vi "4_bit_adder.vi"(0 "A3":bool, 1 "A2":bool, 2 "A1":bool, 3 "A0":bool, 11 "B3":bool, 12 "B2":bool, 13 "B1":bool, 14 "B0":bool) -> (4 "Y4":bool, 6 "Y3":bool, 7 "Somma decimale":dbl, 8 "Y2":bool, 10 "Y1":bool, 15 "Y0":bool)   [LabVIEW 2024]
doc: "Effettua la somma tra 2 numeri binari (di massimo 4 bit ognuno) e ne restituisce la somma in binario e in valore decimale."
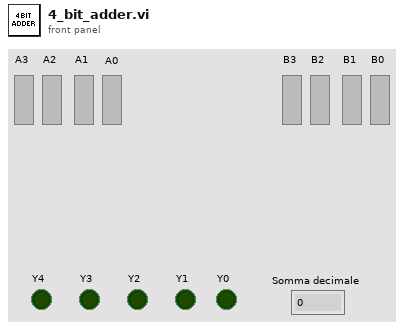
[diagram p1: front panel]
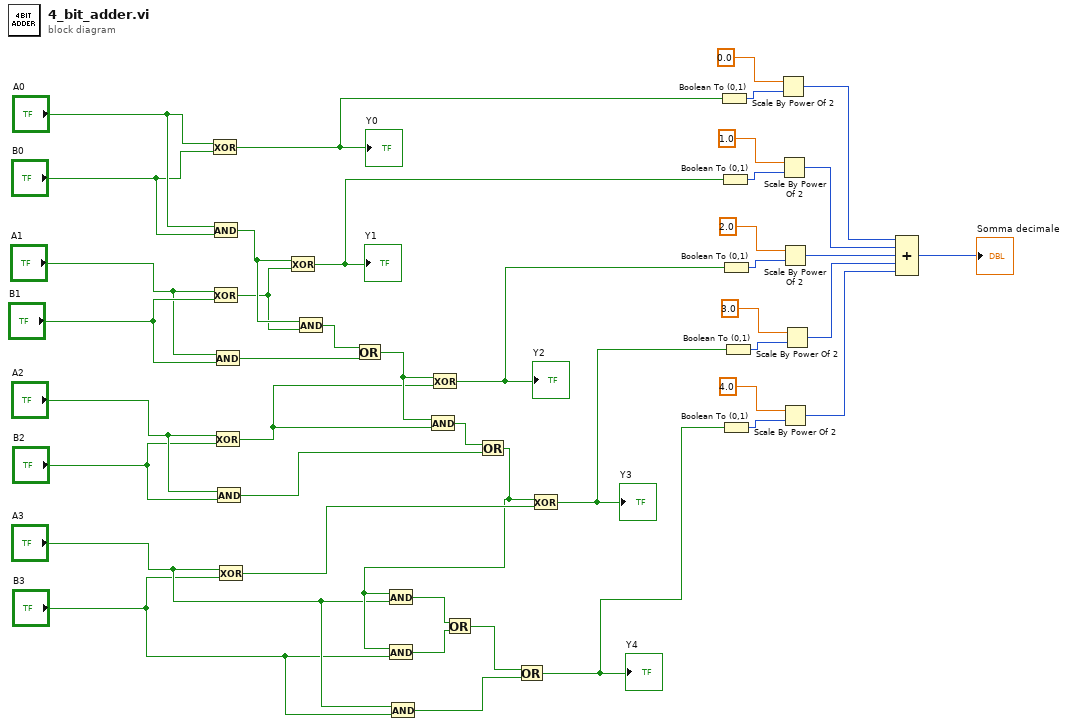
[diagram p0: block diagram]
diagram:
  n1 = Exclusive Or(1:"B0", 2:"A0") -> (0:w5:bool)
  "Y0" <- w5
  n2 = And(x="A0", y="B0") -> (x .and. y?=w39:bool)
  n3 = Exclusive Or(1:"B1", 2:"A1") -> (0:w38:bool)
  n4 = And(x="A1", y="B1") -> (x .and. y?=w37:bool)
  n5 = Exclusive Or(1:"B2", 2:"A2") -> (0:w32:bool)
  n6 = And(x="A2", y="B2") -> (x .and. y?=w30:bool)
  n7 = Exclusive Or(1:"B3", 2:"A3") -> (0:w29:bool)
  n8 = Exclusive Or(1:w38, 2:w39) -> (0:w4:bool)
  "Y1" <- w4
  n9 = And(x=w39, y=w38) -> (x .and. y?=w36:bool)
  n10 = Or(x=w36, y=w37) -> (x .or. y?=w33:bool)
  n11 = And(x="A3", y="B3") -> (x .and. y?=w27:bool)
  n12 = And(x=w33, y=w32) -> (x .and. y?=w31:bool)
  n13 = Exclusive Or(1:w32, 2:w33) -> (0:w3:bool)
  "Y2" <- w3
  n14 = Or(x=w31, y=w30) -> (x .or. y?=w24:bool)
  n15 = And(x=w24, y="A3") -> (x .and. y?=w25:bool)
  n16 = And(x=w24, y="B3") -> (x .and. y?=w26:bool)
  n17 = Or(x=w25, y=w26) -> (x .or. y?=w28:bool)
  n18 = Or(x=w28, y=w27) -> (x .or. y?=w1:bool)
  "Y4" <- w1
  n19 = Exclusive Or(1:w29, 2:w24) -> (0:w2:bool)
  "Y3" <- w2
  n20 = Boolean To (0,1)(Boolean=w5) -> (0, 1=w21:i16)
  n21 = Boolean To (0,1)(Boolean=w4) -> (0, 1=w19:i16)
  n22 = Boolean To (0,1)(Boolean=w3) -> (0, 1=w17:i16)
  n23 = Boolean To (0,1)(Boolean=w1) -> (0, 1=w13:i16)
  n24 = Boolean To (0,1)(Boolean=w2) -> (0, 1=w15:i16)
  n25 = Scale By Power Of 2(n=0.0, x=w21) -> (x*2^n=w9:i16)
  n26 = Scale By Power Of 2(n=1.0, x=w19) -> (x*2^n=w10:i16)
  n27 = Scale By Power Of 2(n=2.0, x=w17) -> (x*2^n=w11:i16)
  n28 = Scale By Power Of 2(n=4.0, x=w13) -> (x*2^n=w7:i16)
  n29 = Scale By Power Of 2(n=3.0, x=w15) -> (x*2^n=w8:i16)
  n30 = Compound Arithmetic op=ADD(w9, w10, w11, w8, w7) -> (→"Somma decimale":i16)
